vi "17.2 Particle Classification-Binary.vi"() -> ()   [LabVIEW 2016]
doc: "This example shows how to use the classification VIs in NI Vision.\n\nClassification quickly identifies and classifies unknown objects in inspection images. First, use the Classification Training Interface to teach your application the types, or classes, of objects you want to classify. The Classification Training Interface creates a classifier file, which you then use to classify unknown objects into one of the classes you trained."
uses:
  <vilib>/vision/NI_Vision_Development_Module.lvlib
panel:
  out "Scores":T1(array[cluster])
  out "Image":T2(plugin-control)
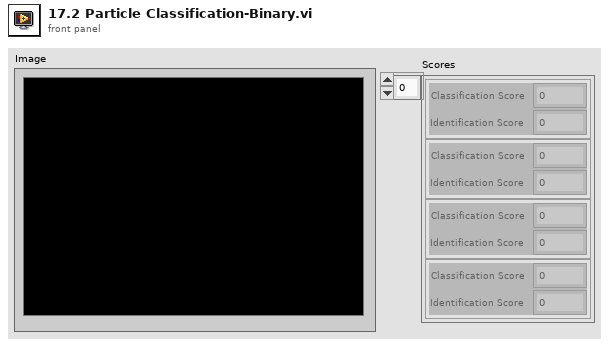
[diagram p1: front panel]
types:
  T1 = cluster{"Classification Score":sgl, "Identification Score":sgl}[]
  T2 = typedef "IMAQ Image.ctl" = refnum<image>
  T3 = typedef "IMAQ Classifier Session.ctl" = refnum<k1>
  T4 = typedef "ROI Descriptor" = cluster{"Global Rectangle":i32[], "Contours":cluster{"ID":enum32{"External", "Internal"}, "Type":u32, "Coordinates":i32[]}[]}
  T5 = cluster{"Classification Score":sgl, "Identification Score":sgl}
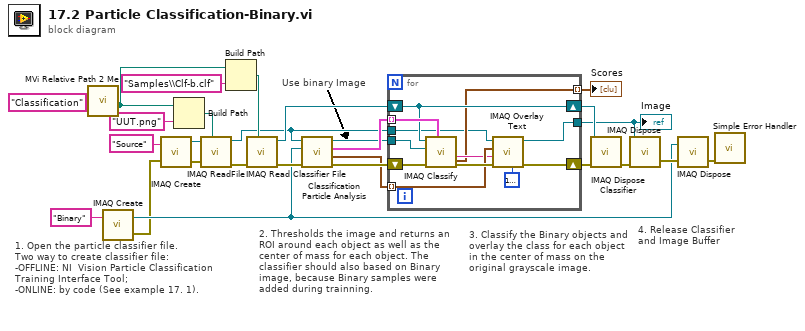
[diagram p0: block diagram]
diagram:
  # "Use binary Image"
  # "4. Release Classifier and Image Buffer"
  # "1. Open the particle classifier file. \nTwo way to create classifier file:\n-OFFLINE: NI  Vision Particle Classification Training Interface Tool;\n-ONLINE: by code (See example 17. 1)."
  # "3. Classify the Binary objects and overlay the class for each object in the center of mass on the original grayscale image."
  # "2. Thresholds the image and returns an ROI around each object as well as the center of mass for each object. The classifier should also based on Binary image, because Binary samples were added during trainning."
  n1 = call "MVi Relative Path 2 Me.vi"("Relative Path"="Classification" ("name or relative path")) -> ("Appended Dir"=w5:path)  [unwired: 5 in, 1 out]
  n2 = call "IMAQ Create"("Image Name"="Binary") -> ("Src"=w12:T2, "error out"=w11:errorcluster)  [unwired: 3 in, 1 out]
  n3 = call "IMAQ Create"("Image Name"="Source", "error in (no error)"=w11) -> ("Src"=w20:T2, "error out"=w19:errorcluster)  [unwired: 2 in, 1 out]
  n4 = Build Path(base path=w5, name or relative path="UUT.png") -> (appended path=w7:path)
  n5 = call "IMAQ ReadFile"("File Path"=w7, "error in (no error)"=w19, "Image"=w20) -> ("error out"=w21:errorcluster, "Image Out"=w1:T2)  [unwired: 4 in, 3 out]
  n6 = Build Path(base path=w5, name or relative path="Samples\\Clf-b.clf") -> (appended path=w22:path)
  n7 = call "IMAQ Read Classifier File"("File Path"=w22, "error in (no error)"=w21) -> ("error out"=w17:errorcluster, "Classifier Session"=w9:T3)  [unwired: 2 in, 6 out]
  n8 = call "Classification Particle Analysis.vi"("error in (no error)"=w17, "Image Dest"=w12, "Image Source"=w1) -> ("error out"=w27:errorcluster, "Center of Masses"=w26:cluster{"X":dbl, "Y":dbl}[], "ROIs"=w25:T4[], "Image Out"=w2:T2)  [unwired: 5 in]
  n9 = for {
    tunnel: w25 -> [w38] mode=indexing
    tunnel: w26 -> [w35] mode=indexing
    shift-right: [w37] -> w16
    shift-left: w9 -> [w37]
    shift-right: [w34] -> w15
    shift-left: w27 -> [w39]
    tunnel: w2 -> [w30]
    tunnel: [w32] -> w4
    tunnel: [w29] -> w3 mode=indexing
    tunnel: w1 -> [w28]
    n10 = call "IMAQ Classify"("ROI Descriptor"=w38, "error in (no error)"=w39, "Image"=w30, "Classifier Session"=w37) -> ("error out"=w36:errorcluster, "Class"=w31:string, "Scores"=w29:T5)  [unwired: 5 out]
    n11 = call "IMAQ Overlay Text"("BG Color (Transparent)"=u32 16777226, "error in (no error)"=w36, "String"=w31, "Origin"=w35, "Image"=w28) -> ("error out"=w34:errorcluster, "Image Out"=w32:T2)  [unwired: 5 in]
  }
  "Image" <- w4
  "Scores" <- w3
  n12 = call "IMAQ Dispose Classifier"("error in (no error)"=w15, "Classifier Session"=w16) -> ("error out"=w14:errorcluster)  [unwired: 9 out]
  n13 = call "IMAQ Dispose"("Image"=w4, "error in (no error)"=w14) -> ("error out"=w13:errorcluster)  [unwired: 1 in, 3 out]
  n14 = call "IMAQ Dispose"("Image"=w12, "error in (no error)"=w13) -> ("error out"=w10:errorcluster)  [unwired: 1 in, 3 out]
  n15 = call <vilib>:"Simple Error Handler.vi"("error in (no error)"=w10) -> ()  [unwired: 4 in, 5 out]
